vi "UE_slave_Create.vi"(8 "error in (no error)":errorcluster, 10 "ID":string, 11 "reference in":refnum<class "UE_slave.lvclass">) -> (0 "error out":errorcluster, 3 "reference out":refnum<class "UE_slave.lvclass">)   [LabVIEW 2019, in "CommandResponse communication.lvlib" / "UE_slave.lvclass"]
doc: "Constructor."
uses:
  UE_slave.lvclass
  C:/Program Files/National Instruments/LabVIEW 2019/vi.lib/addons/_AddQ/G#Object/G#Object.lvclass
  C:/Barkhausen mmWave radar/Development/LV/Barkhausen mmWave hardware control/Host/Intertarget communication/CR slave_class/CR slave.lvclass
  <vilib>/addons/_AddQ/G#Object/G#Object.lvclass
  CR slave_class/CR slave.lvclass
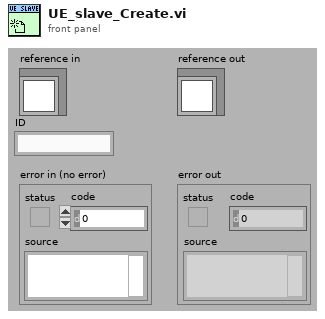
[diagram p1: front panel]
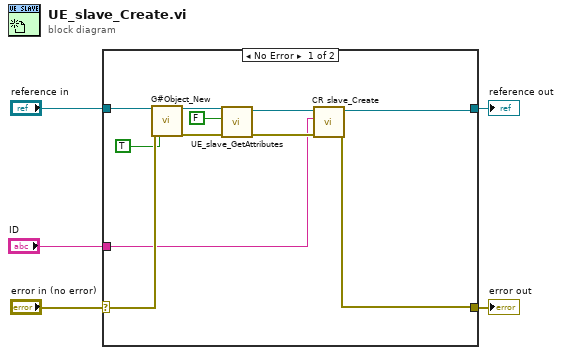
[diagram p0: block diagram]
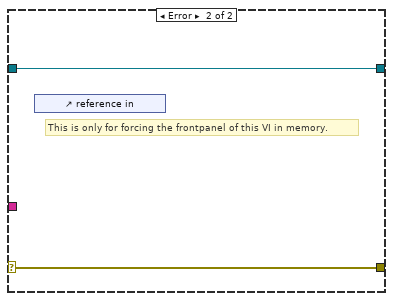
[diagram p2: hidden frame]
diagram:
  n1 = case shown="No Error" "error in (no error)" {
    selector: "error in (no error)" -> [w15 w18]
    tunnel: [w7 w18] -> w4
    tunnel: [w8 w17] -> w2
    tunnel: "reference in" -> [w16 w17]
    tunnel: "ID" -> [w6 _]
    frame No Error {
      n2 = call <vilib>:"G#Object_New.vi"("reference in"=w16, "error in (no error)"=w15, "user counter (T)?"=TRUE ("User Counter")) -> ("reference out"=w11:refnum<class "UE_slave.lvclass">, "error out"=w10:errorcluster)  [unwired: 14 in, 1 out]
      n3 = call "UE_slave_GetAttributes.vi"("error in (no error)"=w10, "return data? (T)"=FALSE ("return data"), "reference in"=w11) -> ("error out"=w13:errorcluster, "reference out"=w9:refnum<class "UE_slave.lvclass">)  [unwired: 5 in, 2 out]
      n4 = call "CR slave_Create.vi"("error in (no error)"=w13, "ID"=w6, "reference in"=w9) -> ("error out"=w7:errorcluster, "reference out"=w8:refnum<class "UE_slave.lvclass">)  [unwired: 7 in]
    }
    frame Error {
      # "This is only for forcing the frontpanel of this VI in memory."
      n5 = control-ref of="reference in"() -> ()  [unwired: 1 out]
    }
  }
  "error out" <- w4
  "reference out" <- w2
